vi "Vision Processing.vi"   [LabVIEW 2013]
doc: "This VI runs in parallel to other tasks. It gets images from the camera, processes them for color or shape and use that information to affect robot behavior."
uses:
  Robot Global Data.vi
types:
  T1 = cluster{"X":dbl, "Y":dbl, "Object":string, "Color":string}[]
  T2 = cluster{"X":dbl, "Y":dbl, "Object":string, "Color":string}
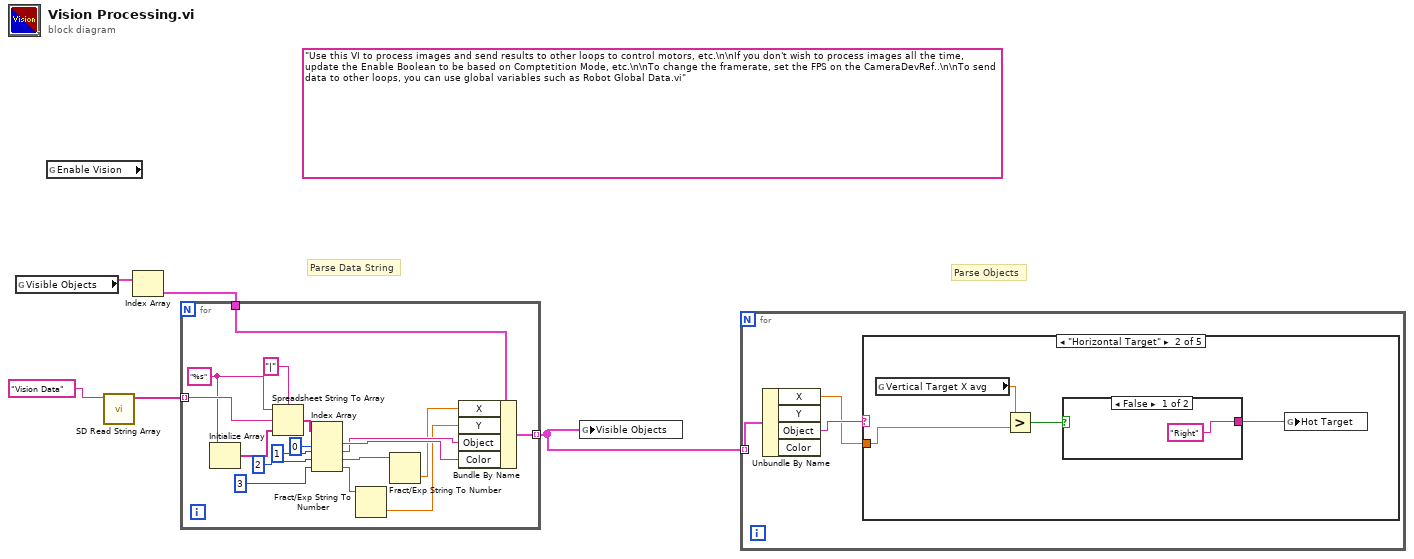
[diagram p0: block diagram]
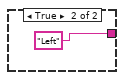
[diagram p3: hidden frame]
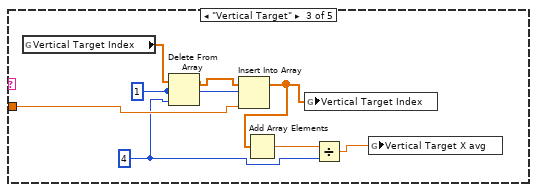
[diagram p4: hidden frame]
diagram:
  (unwired) "Use this VI to process images and send results to other loops to control motors, etc.\n\nIf you don't wish to process images all the time, update the Enable Boolean to be based on Comptetition Mode, etc.\n\nTo change the framerate, set the FPS on the CameraDevRef..\n\nTo send data to other loops, you can use global variables such as Robot Global Data.vi"
  # "Parse Objects"
  # "Parse Data String"
  n1 = global read "Robot Global Data.vi" "Visible Objects"() -> (w3:T1)
  n2 = global read "Robot Global Data.vi" "Enable Vision"() -> ()  [unwired: 1 out]
  n3 = call <vilib>:"SD Read String Array.vi"("Name"="Vision Data") -> ("String Array"=w4:string[])  [unwired: 9 in, 1 out]
  n4 = Index Array(array=w3) -> (element=w2:T2)  [unwired: 1 in]
  n5 = for {
    tunnel: w4 -> [w20] mode=indexing
    tunnel: w2 -> [w22]
    tunnel: [w6] -> w1 mode=indexing
    w18 = "%s"
    n6 = Initialize Array(w18) -> (w19:string[])  [unwired: 1 in]
    n7 = Spreadsheet String To Array(delimiter (Tab)="|", format string=w18, spreadsheet string=w20, array type (2D Dbl)=w19) -> (array=w17:string[])
    n8 = Index Array(array=w17, index #1=0, index #2=1, index #3=2, index #4=3) -> (element #1=w12:string, element #2=w11:string, element #3=w10:string, element #4=w9:string)
    n9 = Fract/Exp String To Number(string=w9) -> (number=w7:dbl)  [unwired: 3 in, 1 out]
    n10 = Fract/Exp String To Number(string=w10) -> (number=w8:dbl)  [unwired: 3 in, 1 out]
    n11 = Bundle By Name(cluster=w22, "X"=w8, "Y"=w7, "Object"=w11, "Color"=w12) -> (w6:T2)
  }
  n12 = global write "Robot Global Data.vi" "Visible Objects"(w1) -> ()
  n13 = for {
    tunnel: w1 -> [w25] mode=indexing
    n14 = Unbundle By Name(w25) -> ("X"=w23:dbl, "Object"=w24:string)  [unwired: 2 out]
    n15 = case shown="\"Horizontal Target\"" w24 {
      tunnel: w23 -> [_ w28 w37 _ _]
      frame "Object", Default {
      }
      frame "Horizontal Target" {
        n16 = global read "Robot Global Data.vi" "Vertical Target X avg"() -> (w29:dbl)
        n17 = Greater?(x=w29, y=w28) -> (0:w27:bool)
        n18 = case shown="False" w27 {
          tunnel: ["Right" "Left"] -> w26
          frame False {
          }
          frame True {
          }
        }
        n19 = global write "Robot Global Data.vi" "Hot Target"(w26) -> ()
      }
      frame "Vertical Target" {
        w35 = 4
        w34 = 1
        n20 = global read "Robot Global Data.vi" "Vertical Target Index"() -> (w39:dbl[])
        n21 = Delete From Array(array=w39, length=w34, index=w35) -> (array with subset deleted=w38:dbl[])  [unwired: 1 out]
        n22 = Insert Into Array(array=w38, index=w34, new element=w37) -> (w33:dbl[])
        n23 = Add Array Elements(numeric array=w33) -> (sum=w36:dbl)
        n24 = global write "Robot Global Data.vi" "Vertical Target Index"(w33) -> ()
        n25 = Divide(x=w36, y=w35) -> (x/y=w32:dbl)
        n26 = global write "Robot Global Data.vi" "Vertical Target X avg"(w32) -> ()
      }
      frame "Ball" {
      }
      frame "Bumper" {
      }
    }
  }
